vi "CS SQL Server.read_ini.vi"() -> (0 "Port":u32)   [LabVIEW 2014, in "CS SQL Server.lvlib"]
doc: "Read TCP/IP socket port from ini-file.\n\n<B>Default:</B> 4711\n\n<B>Hint:</B> Missing data will be added to the ini-file if not found."
uses:
  CS SQL Server.lvlib
  <vilib>/Utility/config.llb/Write Key (U32).vi
  <vilib>/Utility/config.llb/Read Key (U32).vi
  <vilib>/Utility/config.llb/NI_LVConfig.lvlib
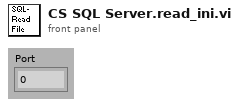
[diagram p1: front panel]
types:
  T1 = enum32{"invalid app kind", "Development System", "Run Time System", "Student Edition", "Embedded LabVIEW", "Evaluation", "Custom"}
  T2 = typedef "NI_LVConfig.lvlib/Config Data RefNum.ctl" = refnum<k1>
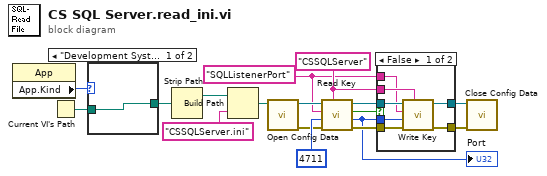
[diagram p0: block diagram]
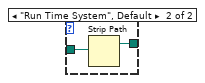
[diagram p2: hidden frame]
diagram:
  w7 = "SQLListenerPort"
  w8 = "CSSQLServer"
  n1 = property class="App"() -> ("App.Kind"=w1:T1)  [unwired: 2 in, 2 out]
  n2 = Current VI's Path() -> (path=w3:path)
  n3 = case shown="\"Development System\"" w1 {
    tunnel: w3 -> [w18 w20]
    tunnel: [w18 w19] -> w2
    frame "Development System" {
    }
    frame "Run Time System", Default {
      n4 = Strip Path(path=w20) -> (stripped path=w19:path)  [unwired: 1 out]
    }
  }
  n5 = Strip Path(path=w2) -> (stripped path=w12:path)  [unwired: 1 out]
  n6 = Build Path(base path=w12, name or relative path="CSSQLServer.ini") -> (appended path=w17:path)
  n7 = call <vilib>:"Open Config Data.vi"("configuration file path"=w17) -> ("error out"=w15:errorcluster, "refnum"=w13:T2)  [unwired: 8 in, 1 out]
  n8 = call-poly <vilib>:"Read Key.vi"("section"=w8, "error in (no error)"=w15, "default value"=u32 4711, "key"=w7, "refnum"=w13) -> ("error out"=w9:errorcluster, "value"=w4:u32, "found?"=w10:bool, "refnum out"=w11:T2)  [unwired: 3 in]
  "Port" <- w4
  n9 = case shown="False" w10 {
    tunnel: w11 -> [w27 w29]
    tunnel: w9 -> [w26 w28]
    tunnel: w8 -> [w25 _]
    tunnel: w7 -> [w24 _]
    tunnel: [w23 w29] -> w6
    tunnel: [w22 w28] -> w5
    tunnel: w4 -> [w21 _]
    frame False {
      n10 = call-poly <vilib>:"Write Key.vi"("section"=w25, "error in (no error)"=w26, "value"=w21, "key"=w24, "refnum"=w27) -> ("error out"=w22:errorcluster, "refnum out"=w23:T2)  [unwired: 4 in, 1 out]
    }
    frame True {
    }
  }
  n11 = call <vilib>:"Close Config Data.vi"("error in (no error)"=w5, "refnum"=w6) -> ()  [unwired: 8 in, 2 out]
